vi "Choose Resource UI.vi"(8 "error in (no error)":errorcluster, 11 "RP2040.lvlib:RP2040Platform in":refnum<class "RP2040Platform.lvclass">) -> (0 "error out":errorcluster, 1 "Cancelled":bool, 2 "Resource":refnum<class "Resource.lvclass">, 3 "RP2040.lvlib:RP2040Platform out":refnum<class "RP2040Platform.lvclass">)   [LabVIEW 2020, in "RP2040.lvlib" / "RP2040Platform.lvclass"]
uses:
  RP2040Platform.lvclass
  Builds/picoG/ppl/PicoG-Core.lvlibp/PicoG-Processor/PicoG-Core/Resource/Resource.lvclass
  RP2040Platform.lvclass/RP2040Platform.ctl
  Builds/picoG/ppl/PicoG-Core.lvlibp/PicoG-Processor/PicoG-Core/SerialResource/SerialResource.lvclass
  C:/dev/picoG/PicoG/Builds/picoG/ppl/PicoG-Core.lvlibp/PicoG-Processor/PicoG-Core/Resource/Resource.lvclass
  C:/dev/picoG/PicoG/Builds/picoG/ppl/PicoG-Core.lvlibp/PicoG-Processor/PicoG-Core/SerialResource/SerialResource.lvclass
panel:
  in  "Resources":i32(listbox)
  in  "Cancel":bool
  in  "OK":bool
  # "Select your RP2040 Resource"
  # "This will reset any app currently running on the device."
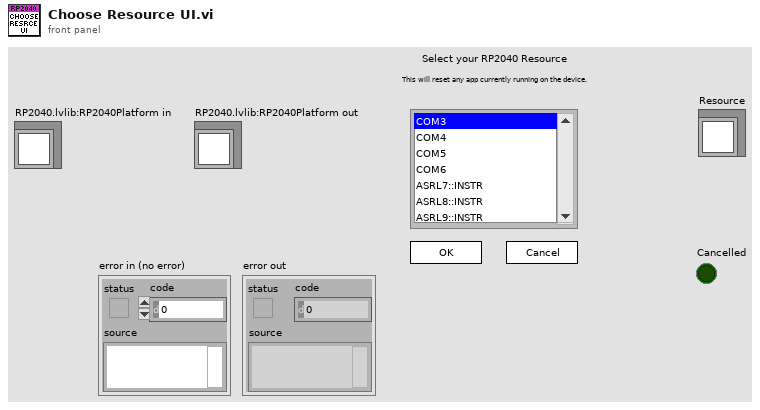
[diagram p1: front panel]
types:
  T1 = enum8{"Enabled", "Disabled", "Disabled and Grayed Out"}
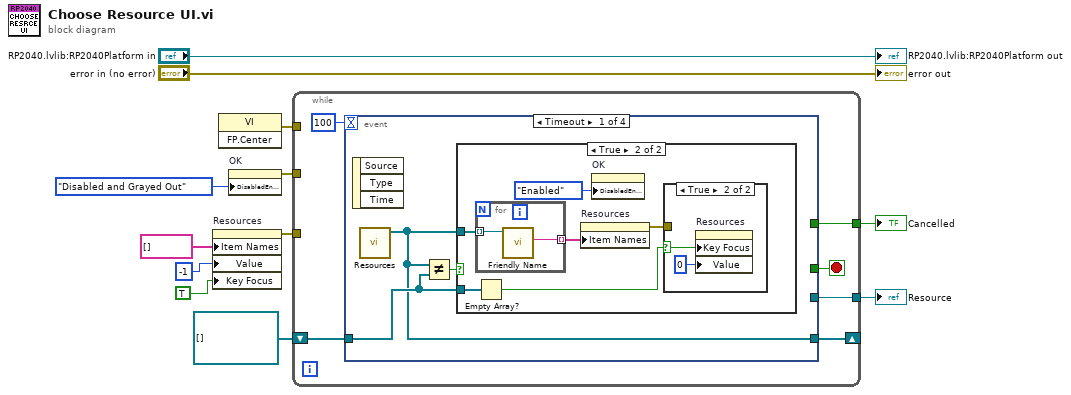
[diagram p0: block diagram]
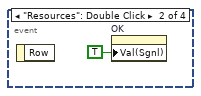
[diagram p4: hidden frame]
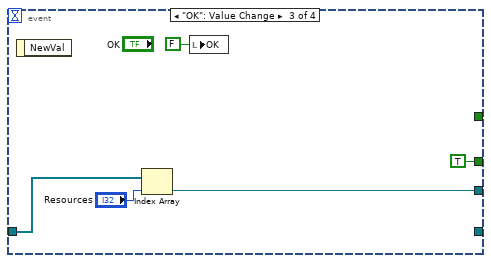
[diagram p5: hidden frame]
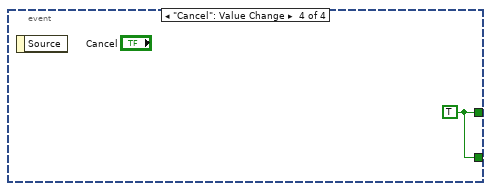
[diagram p6: hidden frame]
diagram:
  n1 = property on="Resources" class="LstBox (strict)"("Item Names"=string[] [], "Value"=-1 ("Resources"), "Key Focus"=TRUE) -> (error out=w3:errorcluster)  [unwired: 2 in, 1 out]
  n2 = invoke class="VI" method="FP.Center"() -> (error out=w1:errorcluster)  [unwired: 3 in, 2 out]
  n3 = property on="OK" class="Bool (strict)"("DisabledEnum"=T1."Disabled and Grayed Out" ("Disabled")) -> (error out=w9:errorcluster)  [unwired: 2 in, 1 out]
  n4 = while {
    shift-right: [w16] -> _
    shift-left: refnum<class "SerialResource.lvclass">[] [] ("Resources") -> [w17]
    tunnel: [w15] -> w11
    tunnel: w9 -> [_]
    tunnel: [w13] -> w4
    tunnel: w3 -> [_]
    tunnel: w1 -> [_]
    stop <- w14 stop-if-true
    n5 = event shown="[0] Timeout" {
      selector: _ -> [_ _ _ _]
      dyn-events: _ -> [_ _ _ _]
      timeout: 100 -> [_ _ _ _]
      tunnel: w17 -> [w20 _ w35 _]
      tunnel: [w19 _ _ _] -> w16
      tunnel: [_ _ _ w38] -> w15
      tunnel: [_ _ TRUE w38] -> w14
      tunnel: [_ _ w34 _] -> w13
      event Timeout {
        n6 = event-data() -> ()  [unwired: 1 in, 3 out]
        n7 = call "Resources.vi"() -> ("Resources"=w19:refnum<class "SerialResource.lvclass">[])  [unwired: 11 in]
        n8 = Not Equal?(x=w19, y=w20) -> (x != y?=w21:bool)
        n9 = case shown="True" w21 {
          tunnel: w20 -> [_ w25]
          tunnel: w19 -> [_ w27]
          frame False {
          }
          frame True {
            n10 = for {
              tunnel: w27 -> [w31] mode=indexing
              tunnel: [w30] -> w26 mode=indexing
              n11 = call-dynamic "Friendly Name.vi"("DeploySerialResource in"=w31) -> ("Friendly Name"=w30:string)  [unwired: 8 in, 2 out]
            }
            n12 = Empty Array?(array=w25) -> (empty?=w23:bool)
            n13 = property on="Resources" class="LstBox (strict)"("Item Names"=w26) -> (error out=w24:errorcluster)  [unwired: 2 in, 1 out]
            n14 = property on="OK" class="Bool (strict)"("DisabledEnum"=T1."Enabled" ("Disabled")) -> ()  [unwired: 2 in, 2 out]
            n15 = case shown="True" w23 {
              selector: w23 -> [_ w29]
              tunnel: w24 -> [_ _]
              frame False {
              }
              frame True {
                n16 = property on="Resources" class="LstBox (strict)"("Key Focus"=w29, "Value"=0 ("Resources")) -> ()  [unwired: 2 in, 2 out]
              }
            }
          }
        }
      }
      event "Resources": Double Click {
        n17 = event-data() -> ()  [unwired: 1 in, 1 out]
        n18 = property on="OK" class="Bool (strict)"("Val(Sgnl)"=TRUE ("Value (Signaling)")) -> ()  [unwired: 2 in, 2 out]
      }
      event "OK": Value Change {
        n19 = event-data() -> ()  [unwired: 1 in, 1 out]
        n20 = Index Array(array=w35, index="Resources") -> (element=w34:refnum<class "SerialResource.lvclass">)
        n21 = local write "OK"(FALSE ("OK")) -> ()
      }
      event "Cancel": Value Change {
        w38 = TRUE
        n22 = event-data() -> ()  [unwired: 1 in, 1 out]
      }
    }
  }
  "Cancelled" <- w11
  "Resource" <- w4
  "error out" <- "error in (no error)"
  "RP2040.lvlib:RP2040Platform out" <- "RP2040.lvlib:RP2040Platform in"
